vi "To Switch Initialization Enum.vi"(11 "initialize and close session behavior":T2) -> (3 "initialization_behavior":T1)   [LabVIEW 2021, in "Session Management niSwitch.lvlib" / "Session Factory.lvclass"]
uses:
  Session Factory.lvclass
  <vilib>/Plug-In SDKs/Sessions/Instrument/ISession Factory/Initialize and Close Session Behavior.ctl
  NI Switch Client/RPC Messages/nidevice_grpc_SessionInitializationBehavior.ctl
  NI Switch Client/NI Switch Client.lvlib
  <vilib>/Plug-In SDKs/Sessions/Instrument/ISession Factory/ISession Factory.lvclass
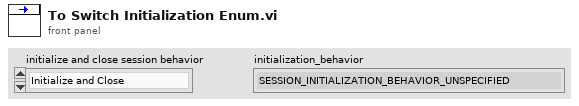
[diagram p1: front panel]
types:
  T1 = typedef "NI Switch Client.lvlib/nidevice_grpc_SessionInitializationBehavior.ctl" = enum32{"SESSION_INITIALIZATION_BEHAVIOR_UNSPECIFIED", "SESSION_INITIALIZATION_BEHAVIOR_INITIALIZE_NEW", "SESSION_INITIALIZATION_BEHAVIOR_ATTACH_TO_EXISTING"}
  T2 = typedef "NI Session Management Instrument.lvlib/ISession Factory.lvclass/Initialize and Close Session Behavior.ctl" = enum16{"Initialize and Close", "Attach and Detach", "Initialize and Detach", "Attach and Close"}
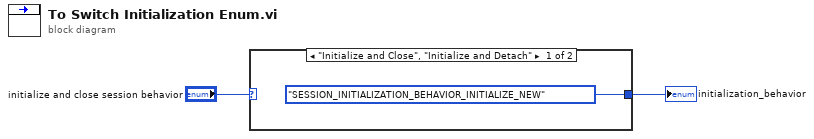
[diagram p0: block diagram]
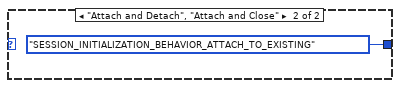
[diagram p2: hidden frame]
diagram:
  n1 = case shown="\"Initialize and Close\", \"Initialize and Detach\"" "initialize and close session behavior" {
    tunnel: [nidevice_grpc_SessionInitializationBehavior."SESSION_INITIALIZATION_BEHAVIOR_INITIALIZE_NEW" ("initialization_behavior") nidevice_grpc_SessionInitializationBehavior."SESSION_INITIALIZATION_BEHAVIOR_ATTACH_TO_EXISTING" ("initialization_behavior")] -> w1
    frame "Initialize and Close", "Initialize and Detach" {
    }
    frame "Attach and Detach", "Attach and Close" {
    }
  }
  "initialization_behavior" <- w1
